vi "señ.vi"(10 "Orden":T2(array[ring]), 11 "Enum":T1(ring)) -> (1 "element":T1(ring))   [LabVIEW 2016]
doc: "Indica el siguiente elemento que se tendría que ejecutar de acuerdo al orden que asignó el usuario.\n\nLas entradas son:\nEl arreglo de orden en el que se tienen que ejecutar los elementos.\nTambién entra el estado actual en el que se encuentra en la maquina de estados.\n\nComo salida tiene el siguiente elemento."
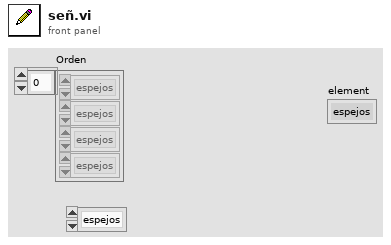
[diagram p1: front panel]
types:
  T1 = enum16{"espejos", "polarizador", "voltaje", "potenciometro y lockin", "CCD"}
  T2 = enum16{"espejos", "polarizador", "voltaje", "potenciometro y lockin", "CCD"}[]
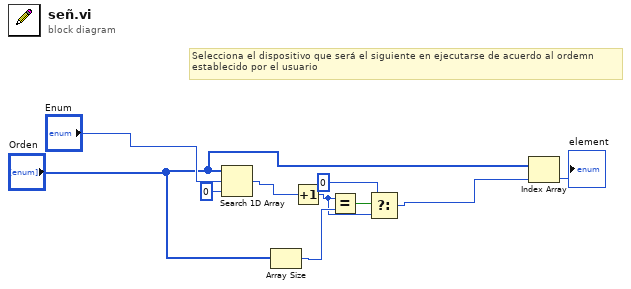
[diagram p0: block diagram]
diagram:
  # "Selecciona el dispositivo que será el siguiente en ejecutarse de acuerdo al ordemn\nestablecido por el usuario"
  n1 = Search 1D Array(1D array="Orden", element="Enum", start index (0)=0) -> (index of element=w9:i32)
  n2 = Array Size(array="Orden") -> (size(s)=w8:i32)
  n3 = Increment(x=w9) -> (x+1=w6:i32)
  n4 = Equal?(x=w6, y=w8) -> (x = y?=w7:bool)
  n5 = Select(t=0, s=w7, f=w6) -> (s? t:f=w4:i32)
  n6 = Index Array(array="Orden", index=w4) -> (element=→"element":T1)
